vi "MovePortToEnd.vi"(8 "error in (no error)":errorcluster) -> (0 "error out":errorcluster)   [LabVIEW 2015]
uses:
  Framework/Robot Global Data.vi
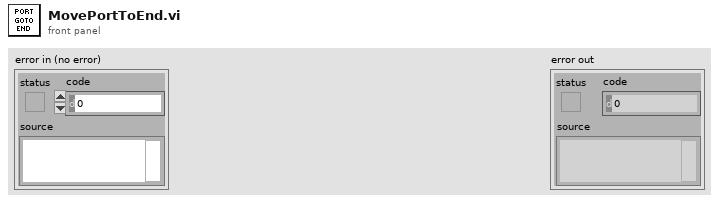
[diagram p1: front panel]
types:
  T1 = typedef "PortC Arm Settings Type Def.ctl" = cluster{"Start Position":dbl, "Down Position":dbl}
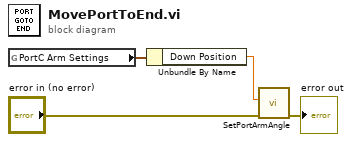
[diagram p0: block diagram]
diagram:
  n1 = global read "Robot Global Data.vi" "PortC Arm Settings"() -> (w4:T1)
  n2 = Unbundle By Name(w4) -> ("Down Position"=w3:dbl)
  n3 = call "SetPortArmAngle.vi"("error in (no error)"="error in (no error)", "Ticks"=w3) -> ("error out"=→"error out":errorcluster)  [unwired: 9 in]
